vi "Load Subroutine Test Exec.vi"(4 "Path Builder":refnum<class "IPath Builder.lvclass">, 5 "Subroutine in":refnum<class "Subroutine.lvclass">, 6 "Persistence in":refnum<class "IPersist.lvclass">, 7 "Linked List ID":string, 8 "error in (no error)":errorcluster, 10 "Subroutine Path":path, 11 "Linked List Ref":refnum<data-value>) -> (0 "error out":errorcluster, 1 "Test File Version Match":bool, 2 "Test Executive Version Match":bool, 3 "Linked List Ref out":refnum<data-value>)   [LabVIEW 2017, in "Test Executive.lvlib" / "Subroutine.lvclass"]
uses:
  <vilib>/gpm_packages/@cs/test-executive/Source/Test Executive/Subroutine/Subroutine.lvclass
  <vilib>/gpm_packages/@cs/linked-list/Source/Linked List/ILinkedList/ILinked List.lvclass
  <vilib>/gpm_packages/@cs/persistence/source/IPersist/IPersist.lvclass
  <vilib>/gpm_packages/@cs/test-executive/Source/Path Builder/IPath Builder/IPath Builder.lvclass
  <vilib>/gpm_packages/@cs/test-executive/Source/Test Executive/ITestExecutive/ITest Executive.lvclass
  <vilib>/gpm_packages/@cs/test-executive/Source/Test Executive/TestExecutive/Test Executive.lvclass
  C:/Program Files/National Instruments/LabVIEW 2017/vi.lib/gpm_packages/@cs/test-executive/Source/Test Executive/ITestExecutive/ITest Executive.lvclass
  99eec8f0-50ee-49f4-9012-2cedafc9663f.vi
  52bac3b5-23a8-4328-aead-fdf0a8238b8f.vi
  4a0ddc4e-31ac-45dd-9084-e524783595b4.vi
  7ffadc8e-1916-414d-bbdc-0be25d1b259b.vi
  448d75c9-5150-43a6-92ed-3c4cd4604ddf.vi
  49529079-acff-4e9f-a028-20bc5060d501.vi
  af76f34b-2ebe-473d-a8fe-d81e58e65588.vi
  ddc1e080-61ae-45a4-a330-8d8f04fba54d.vi
  <vilib>/Utility/error.llb/Error Cluster From Error Code.vi
  <vilib>/gpm_packages/@cs/test-executive/Source/Test Executive/TestExecutive Ref/TestExecutive Ref.lvclass
  <vilib>/gpm_packages/@cs/linked-list/Source/Linked List/Linked List Ref/Linked List Ref.lvclass
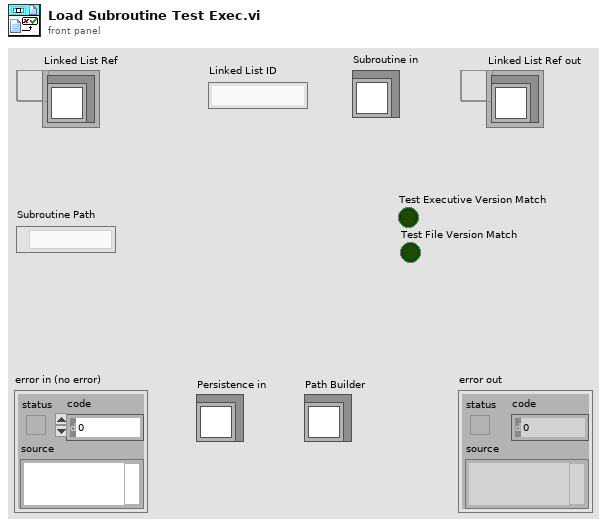
[diagram p1: front panel]
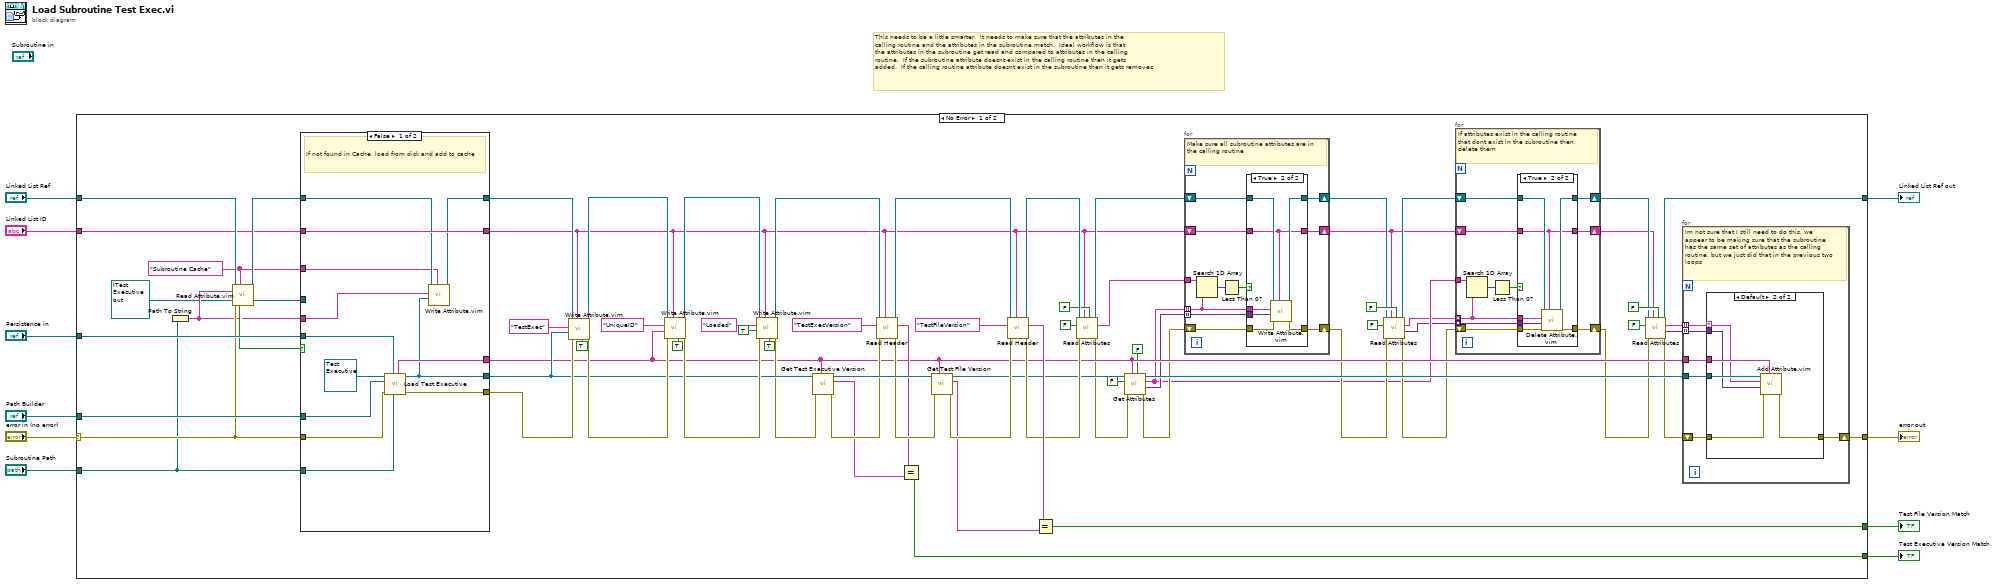
[diagram p0: block diagram]
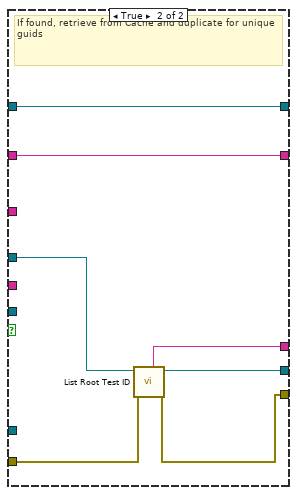
[diagram p2: hidden frame]
diagram:
  # "This needs to be a little smarter.  It needs to make sure that the attributes in the\ncalling routine and the attributes in the subroutine match.  Ideal workflow is that\nthe attributes in the subroutine get read and compared to attributes in the calling\nroutine.  If the subroutine attribute doesnt exist in the calling routine then it gets \nadded.  If the calling routine attribute doesnt exist in the subroutine then it gets removec"
  n1 = case shown="No Error" "error in (no error)" {
    selector: "error in (no error)" -> [w21 w162]
    tunnel: "Persistence in" -> [w76 _]
    tunnel: "Subroutine Path" -> [w20 _]
    tunnel: "Path Builder" -> [w75 _]
    tunnel: "Linked List Ref" -> [w22 w163]
    tunnel: [w58 _] -> w5
    tunnel: [w57 _] -> w4
    tunnel: "Linked List ID" -> [w16 _]
    tunnel: [w28 w163] -> w2
    tunnel: [w53 w162] -> w1
    frame No Error {
      w13 = "Subroutine Cache" ("Name")
      n2 = Path To String(path=w20) -> (string=w14:string)
      n3 = call "Read Attribute.vim"("Linked List Ref"=w22, "Linked List ID"=w13, "Attribute Name"=w14, "Type"=refnum<data-value> refnum ("Test Executive Ref out"), "error in (no error)"=w21) -> ("Linked List Ref out"=w18:refnum<data-value>, "Attribute"=w11:refnum<data-value>, "Found?"=w19:bool)  [unwired: 5 in, 3 out]
      n4 = case shown="False" w19 {
        tunnel: [w98 w103] -> w82
        tunnel: w76 -> [w97 _]
        tunnel: w75 -> [w96 _]
        tunnel: [w87 w101] -> w72
        tunnel: [w88 w100] -> w49
        tunnel: w21 -> [w95 w104]
        tunnel: w20 -> [w94 _]
        tunnel: [w91 w106] -> w17
        tunnel: w18 -> [w92 w106]
        tunnel: [w93 w105] -> w15
        tunnel: w16 -> [w93 w105]
        tunnel: w14 -> [w89 _]
        tunnel: w13 -> [w90 _]
        tunnel: w11 -> [_ w102]
        frame False {
          # "If not found in Cache, load from disk and add to cache"
          n5 = call <vilib>:"Load Test Executive.vi"("Folder"=w94, "Persistence in"=w97, "error in (no error)"=w95, "Path Builder"=w96, "Test Executive"=refnum<class "Test Executive.lvclass"> refnum ("Test Executive.lvlib:Test Executive.lvclass")) -> ("error out"=w98:errorcluster, "Test Executive Ref out"=w87:refnum<data-value>, "Root ID"=w88:string)  [unwired: 4 in]
          n6 = call "Write Attribute.vim"("Linked List ID"=w90, "Attribute"=w87, "Attribute Name"=w89, "Linked List Ref"=w92) -> ("Linked List Ref out"=w91:refnum<data-value>)  [unwired: 4 in, 3 out]
        }
        frame True {
          # "If found, retrieve from Cache and duplicate for unique guids"
          n7 = call <vilib>:"List Root Test ID.vi"("error in (no error)"=w104, "Test Executive Ref"=w102) -> ("error out"=w103:errorcluster, "Test Executive Ref out"=w101:refnum<data-value>, "Root ID"=w100:string)  [unwired: 5 in, 2 out]
        }
      }
      n8 = call "Write Attribute.vim"("Private?"=TRUE, "Linked List ID"=w15, "error in (no error)"=w82, "Attribute"=w72, "Attribute Name"="TestExec", "Linked List Ref"=w17) -> ("error out"=w83:errorcluster, "Linked List Ref out"=w74:refnum<data-value>)  [unwired: 2 in, 2 out]
      n9 = call "Write Attribute.vim"("Private?"=TRUE, "Linked List ID"=w15, "error in (no error)"=w83, "Attribute"=w49, "Attribute Name"="UniqueID", "Linked List Ref"=w74) -> ("error out"=w78:errorcluster, "Linked List Ref out"=w73:refnum<data-value>)  [unwired: 2 in, 2 out]
      n10 = call "Write Attribute.vim"("Private?"=TRUE, "Linked List ID"=w15, "error in (no error)"=w78, "Attribute"=TRUE, "Attribute Name"="Loaded", "Linked List Ref"=w73) -> ("error out"=w70:errorcluster, "Linked List Ref out"=w69:refnum<data-value>)  [unwired: 2 in, 2 out]
      n11 = call <vilib>:"Get Test Executive Version.vi"("Unique ID"=w49, "error in (no error)"=w70, "Test Executive Ref"=w72) -> ("error out"=w67:errorcluster, "Test Executive Version"=w61:string, "Test Executive Ref out"=w71:refnum<data-value>)  [unwired: 5 in, 1 out]
      n12 = call <vilib>:"Read Header.vi"("Linked List ID"=w15, "error in (no error)"=w67, "Header Name"="TestExecVersion" ("String"), "Linked List Ref"=w69) -> ("error out"=w66:errorcluster, "Header Value"=w62:string, "Linked List Ref out"=w65:refnum<data-value>)  [unwired: 4 in, 1 out]
      n13 = Equal?(x=w62, y=w61) -> (x = y?=w58:bool)
      n14 = call <vilib>:"Get Test File Version.vi"("Unique ID"=w49, "error in (no error)"=w66, "Test Executive Ref"=w71) -> ("error out"=w64:errorcluster, "Test File Version"=w59:string, "Test Executive Ref out"=w51:refnum<data-value>)  [unwired: 5 in, 1 out]
      n15 = call <vilib>:"Read Header.vi"("Linked List ID"=w15, "error in (no error)"=w64, "Header Name"="TestFileVersion" ("String"), "Linked List Ref"=w65) -> ("error out"=w55:errorcluster, "Header Value"=w60:string, "Linked List Ref out"=w56:refnum<data-value>)  [unwired: 4 in, 1 out]
      n16 = Equal?(x=w60, y=w59) -> (x = y?=w57:bool)
      n17 = call <vilib>:"Read Attributes.vi"("Flatten Pointer?"=FALSE, "Linked List ID"=w15, "error in (no error)"=w55, "Include Private?"=FALSE, "Linked List Ref"=w56) -> ("error out"=w46:errorcluster, "Attribute Names out"=w45:string[], "Linked List Ref out"=w43:refnum<data-value>)  [unwired: 1 in, 3 out]
      n18 = call <vilib>:"Get Attributes.vi"("Flatten Pointer?"=FALSE, "Test ID"=w49, "error in (no error)"=w46, "Include Private?"=FALSE, "Test Executive Ref"=w51) -> ("error out"=w42:errorcluster, "Attributes"=w44:variant[], "Attribute Names out"=w34:string[], "Test Executive Ref out"=w50:refnum<data-value>)  [unwired: 1 in, 2 out]
      n19 = for {
        tunnel: w34 -> [w130] mode=indexing
        tunnel: w44 -> [w129] mode=indexing
        shift-right: [w135] -> w38
        shift-left: w43 -> [w136]
        tunnel: w45 -> [w137]
        shift-right: [w133] -> w39
        shift-left: w42 -> [w134]
        shift-right: [w128] -> w36
        shift-left: w15 -> [w132]
        # "Make sure all subroutine attributes are in the calling routine"
        n20 = Search 1D Array(1D array=w137, element=w130) -> (index of element=w138:i32)  [unwired: 1 in]
        n21 = Less Than 0?(x=w138) -> (x < 0?=w131:bool)
        n22 = case shown="True" w131 {
          tunnel: w136 -> [w141 w148]
          tunnel: [w141 w147] -> w135
          tunnel: w134 -> [w140 w146]
          tunnel: [w140 w145] -> w133
          tunnel: w132 -> [w139 w142]
          tunnel: w130 -> [_ w144]
          tunnel: w129 -> [_ w143]
          tunnel: [w139 w142] -> w128
          frame False {
          }
          frame True {
            n23 = call "Write Attribute.vim"("Linked List ID"=w142, "error in (no error)"=w146, "Attribute"=w143, "Attribute Name"=w144, "Linked List Ref"=w148) -> ("error out"=w145:errorcluster, "Linked List Ref out"=w147:refnum<data-value>)  [unwired: 3 in, 2 out]
          }
        }
      }
      n24 = call <vilib>:"Read Attributes.vi"("Flatten Pointer?"=FALSE, "Linked List ID"=w36, "error in (no error)"=w39, "Include Private?"=FALSE, "Linked List Ref"=w38) -> ("error out"=w35:errorcluster, "Attributes"=w32:variant[], "Attribute Names out"=w33:string[], "Linked List Ref out"=w37:refnum<data-value>)  [unwired: 1 in, 2 out]
      n25 = for {
        tunnel: w33 -> [w109] mode=indexing
        tunnel: w32 -> [w108] mode=indexing
        shift-right: [w114] -> w29
        shift-left: w37 -> [w115]
        tunnel: w34 -> [w116]
        shift-right: [w112] -> w26
        shift-left: w35 -> [w113]
        shift-right: [w107] -> w27
        shift-left: w36 -> [w111]
        # "If attributes exist in the calling routine that dont exist in the subroutine then delete them"
        n26 = Search 1D Array(1D array=w116, element=w109) -> (index of element=w117:i32)  [unwired: 1 in]
        n27 = Less Than 0?(x=w117) -> (x < 0?=w110:bool)
        n28 = case shown="True" w110 {
          tunnel: w115 -> [w120 w127]
          tunnel: [w120 w126] -> w114
          tunnel: w113 -> [w119 w124]
          tunnel: [w119 w123] -> w112
          tunnel: w111 -> [w118 w125]
          tunnel: w109 -> [_ w122]
          tunnel: w108 -> [_ w121]
          tunnel: [w118 w125] -> w107
          frame False {
          }
          frame True {
            n29 = call "Delete Attribute.vim"("Linked List ID"=w125, "error in (no error)"=w124, "Type"=w121, "Attribute Name"=w122, "Linked List Ref"=w127) -> ("error out"=w123:errorcluster, "Linked List Ref out"=w126:refnum<data-value>)  [unwired: 4 in, 1 out]
          }
        }
      }
      n30 = call <vilib>:"Read Attributes.vi"("Flatten Pointer?"=FALSE, "Linked List ID"=w27, "error in (no error)"=w26, "Include Private?"=FALSE, "Linked List Ref"=w29) -> ("error out"=w25:errorcluster, "Attributes"=w24:variant[], "Attribute Names out"=w23:string[], "Linked List Ref out"=w28:refnum<data-value>)  [unwired: 1 in, 2 out]
      n31 = for {
        tunnel: w50 -> [w154]
        tunnel: w49 -> [w153]
        shift-right: [w151] -> w53
        shift-left: w25 -> [w152]
        tunnel: w23 -> [w150] mode=indexing
        tunnel: w24 -> [w149] mode=indexing
        # "Im not sure that I still need to do this, we appear to be making sure that the subroutine has the same set of attributes as the calling routine, but we just did that in the previous two loops"
        n32 = case shown="Default" w150 {
          selector: w150 -> [_ w157]
          tunnel: w154 -> [_ w161]
          tunnel: w153 -> [_ w160]
          tunnel: w152 -> [w155 w159]
          tunnel: [w155 w158] -> w151
          tunnel: w149 -> [_ w156]
          frame "Restore Point" {
          }
          frame Default {
            n33 = call "Add Attribute.vim"("ID"=w160, "error in (no error)"=w159, "Attribute"=w156, "Attribute Name"=w157, "Test Executive Ref"=w161) -> ("error out"=w158:errorcluster)  [unwired: 3 in, 3 out]
          }
        }
      }
    }
    frame Error {
    }
  }
  "error out" <- w1
  "Linked List Ref out" <- w2
  "Test Executive Version Match" <- w5
  "Test File Version Match" <- w4
